vi "Defender_din_lorero.vi"(8 "IA State":T7={"our_robots"=[], "enemy_robots"=[], "balls"=[], "geometry"={"field_length"=0, "field_width"=0, "goal_width"=0, "goal_depth"=0, "center_circle_radius"=0, "defense_width"=0, "defense_depth"=0, "free_kick_from_defense_dist"=0, "penalty_spot_from_field_line_dist"=0, "penalty_line_from_spot_dist"=0, "half_moon_depth"=0, "half_moon_width"=0}, "IA Judge"={"stage"="", "command"="", "our_goalie_id"=0.0, "enemy_goalie_id"=0.0, "command enum"=enum."Halt", "Time"=enum."Azul"}, "Received Timestamp"=timestamp(0 s since 1904-01-01), "Events"={"Touch"=FALSE, "id touch"=0.0, "Ball out of \nVision"=FALSE, "Ball inside \nGoalie area"=FALSE, "Robot not responding"=FALSE, "Robots responding status"=[1.0, 1.0, 1.0, 1.0, 1.0, 1.0], "Enemy Ball \nPossession"=FALSE, "Id ini Possession"=0.0, "Ball Possesion"=FALSE, "Id Possesion"=0.0, "Ball at\nour goal side"=FALSE, "Ball at\ntouchline"=FALSE, "Ball at\nenemy goal side"=FALSE}}, 10 "balls":T6[](array[typedef]), 11 "Robot in":T1) -> (1 "Robot out":T1)   [LabVIEW 2018]
uses:
  Core/AI Robot.ctl
  Functions Enum.ctl
  AttackerStates.ctl
  Path Planning/RRT/PathDests.ctl
  Path Planning/RRT/PathDest.ctl
  Core/AI Input.ctl
  Core/AI Ball.ctl
  Core/Field Size.ctl
  Core/AI Judge.ctl
  Command Enum.ctl
  Util/Events/Events.ctl
  <vilib>/Analysis/_algsub.llb/Real Vector Norm.vi
  <vilib>/Analysis/NI_AALPro.lvlib
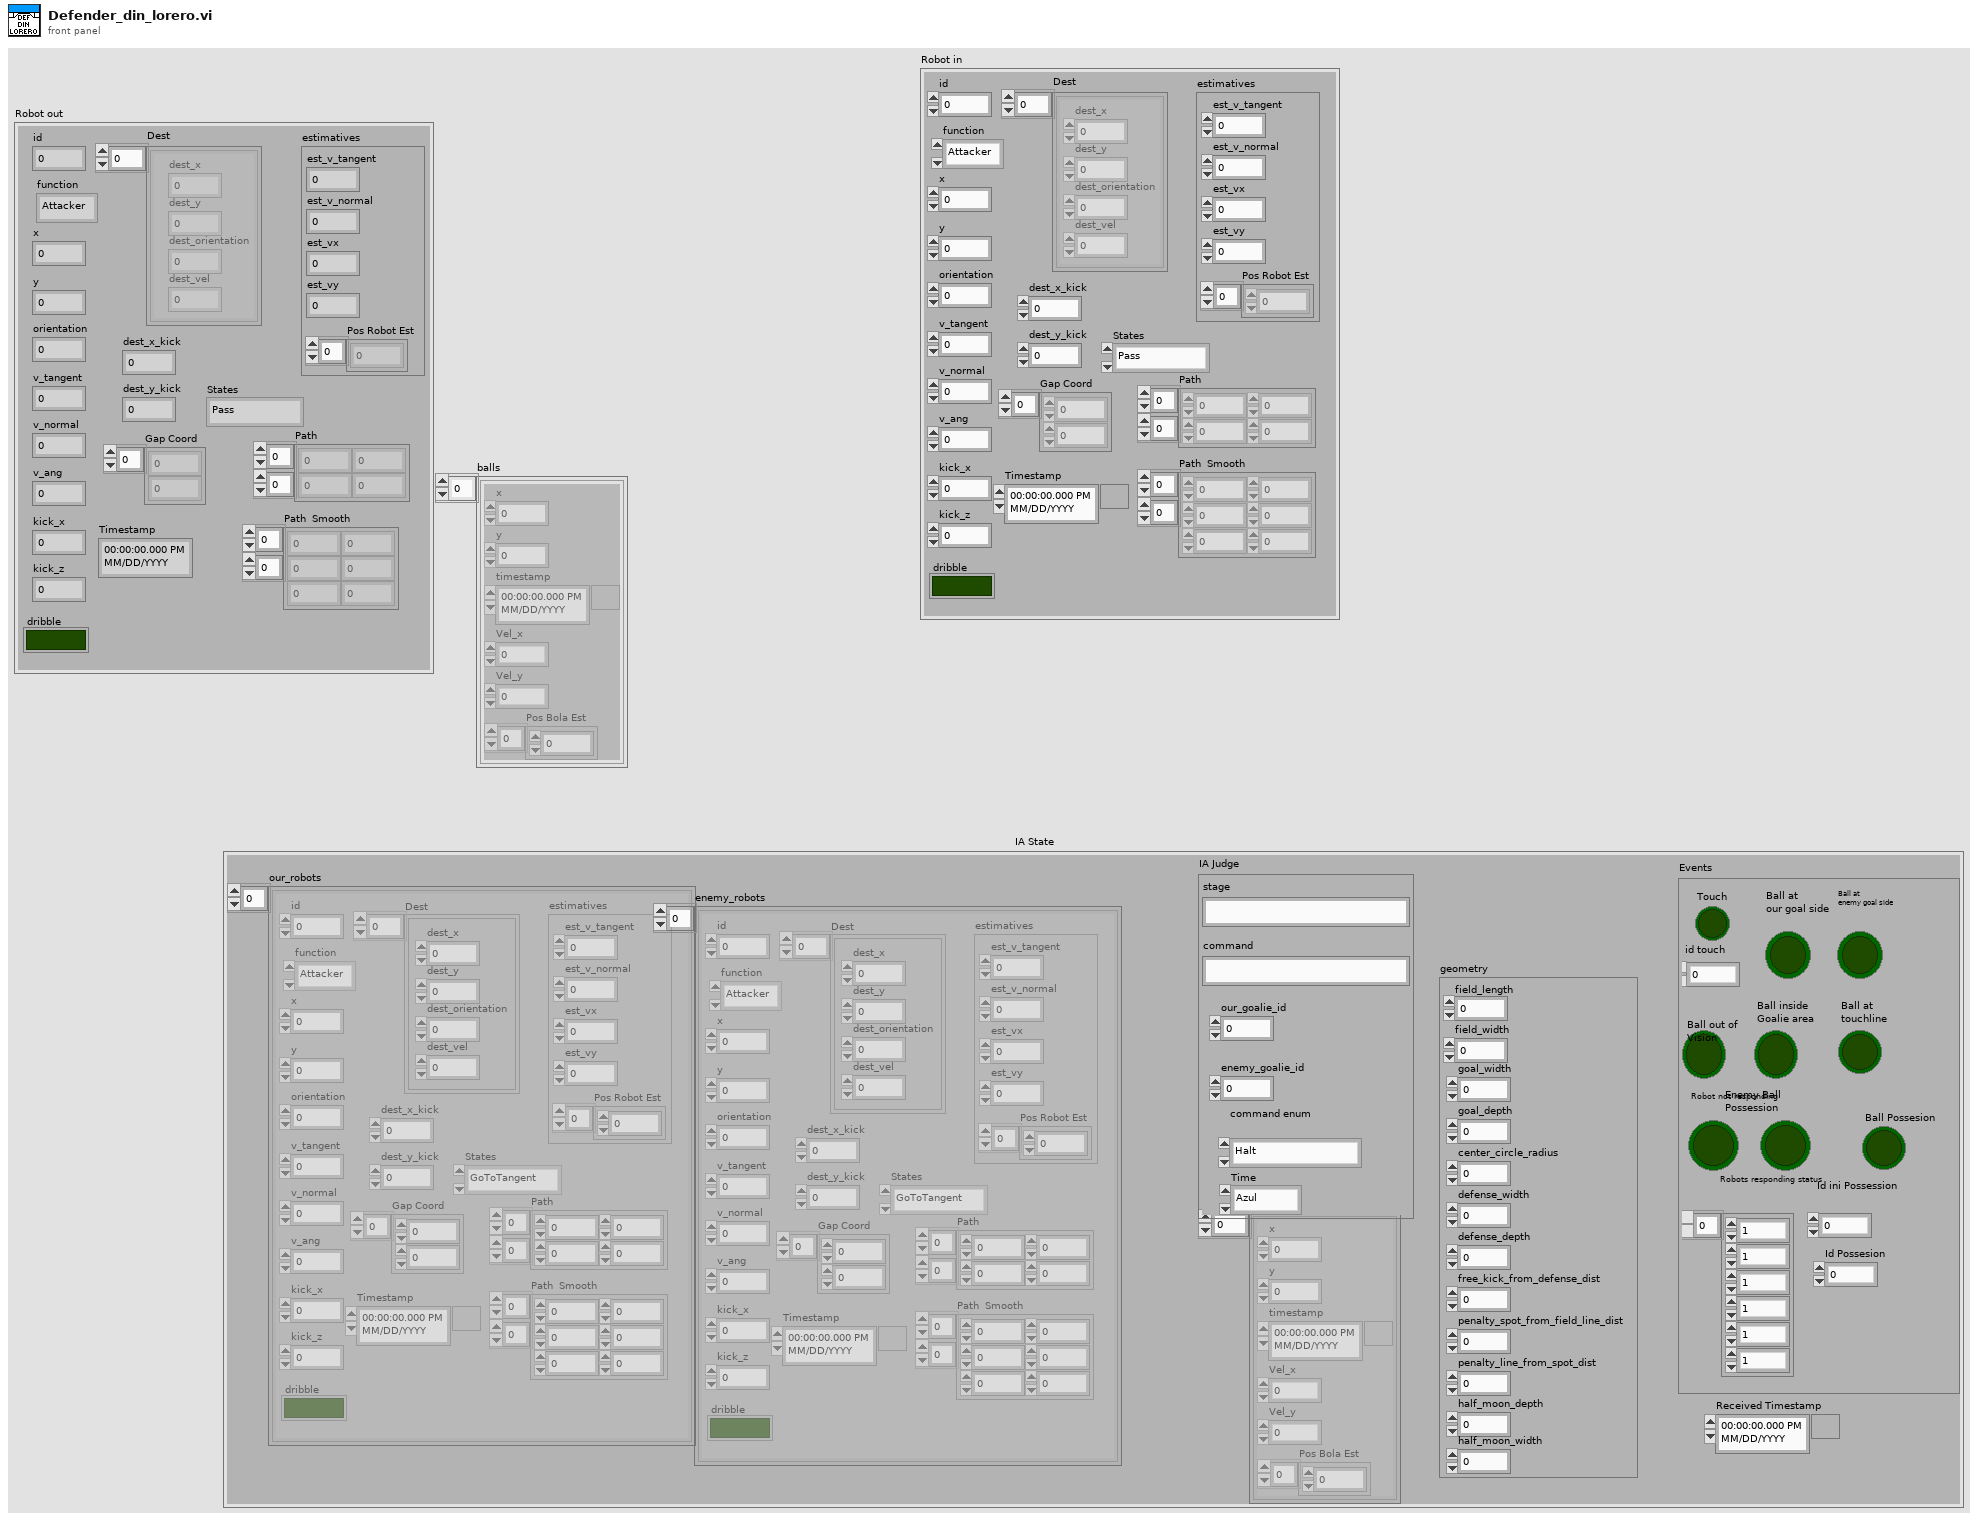
[diagram p1: front panel]
types:
  T1 = typedef "AI Robot.ctl" = cluster{"id":u32, "function":T2, "x":dbl, "y":dbl, "orientation":dbl, "v_tangent":dbl, "v_normal":dbl, "v_ang":dbl, "kick_x":dbl, "kick_z":dbl, "dribble":bool, "Timestamp":timestamp, "estimatives":cluster{"est_v_tangent":dbl, "est_v_normal":dbl, "est_vx":dbl, "est_vy":dbl, "Pos Robot Est":dbl[]}, "dest_x_kick":dbl, "dest_y_kick":dbl, "Gap Coord":dbl[], "States":T3, "Path ":dbl[][], "Path  Smooth":dbl[][], "Dest":T4}
  T2 = typedef "Functions Enum.ctl" = enum16{"Attacker", "Goalie", "Defender", "Striker", "Goto 0", "Dummy", "Kicker", "ZigZag"}
  T3 = typedef "AttackerStates.ctl" = enum16{"Pass", "GoToTangent", "BallGetting", "GoToKick", "Rotate anti-clockwise", "Rotate Clockwise", ""}
  T4 = typedef "PathDests.ctl" = T5[]
  T5 = typedef "PathDest.ctl" = cluster{"dest_x":dbl, "dest_y":dbl, "dest_orientation":dbl, "dest_vel":dbl}
  T6 = typedef "AI Ball.ctl" = cluster{"x":dbl, "y":dbl, "timestamp":timestamp, "Vel_x":dbl, "Vel_y":dbl, "Pos Bola Est":dbl[]}
  T7 = typedef "AI Input.ctl" = cluster{"our_robots":T1[], "enemy_robots":T1[], "balls":T6[], "geometry":T8, "IA Judge":T9, "Received Timestamp":timestamp, "Events":T11}
  T8 = typedef "Field Size.ctl" = cluster{"field_length":u32, "field_width":u32, "goal_width":u32, "goal_depth":u32, "center_circle_radius":u32, "defense_width":u32, "defense_depth":u32, "free_kick_from_defense_dist":u32, "penalty_spot_from_field_line_dist":u32, "penalty_line_from_spot_dist":u32, "half_moon_depth":u32, "half_moon_width":u32}
  T9 = typedef "AI Judge.ctl" = cluster{"stage":string, "command":string, "our_goalie_id":dbl, "enemy_goalie_id":dbl, "command enum":T10, "Time":enum16{"Azul", "Amarelo"}}
  T10 = typedef "Command Enum.ctl" = enum16{"Halt", "Stop", "Force Start", "PKA Normal Start", "Prepare Kickoff Ally", "PKE Normal Start", "Prepare Kickoff Enemy", "Prepare Penalty Ally", "PPA Normal Start", "Prepare Penalty Enemy", "PPE Normal Start", "Ball Placement Enemy Up", "Ball Placement Enemy Down", "Ball Placement Ally Up", "Ball Placement Ally Mid", "Ball Placement Ally Down", "Indirect Free Enemy", "Indirect Free Ally", "Timeout Enemy", "Timeout Ally", "Goal Enemy", "Goal Ally", "Normal Half Time", "Extra Time Break", "Extra Half Time", "None", "Post Game"}
  T11 = typedef "Events.ctl" = cluster{"Touch":bool, "id touch":dbl, "Ball out of \nVision":bool, "Ball inside \nGoalie area":bool, "Robot not responding":bool, "Robots responding status":dbl[], "Enemy Ball \nPossession":bool, "Id ini Possession":dbl, "Ball Possesion":bool, "Id Possesion":dbl, "Ball at\nour goal side":bool, "Ball at\ntouchline":bool, "Ball at\nenemy goal side":bool}
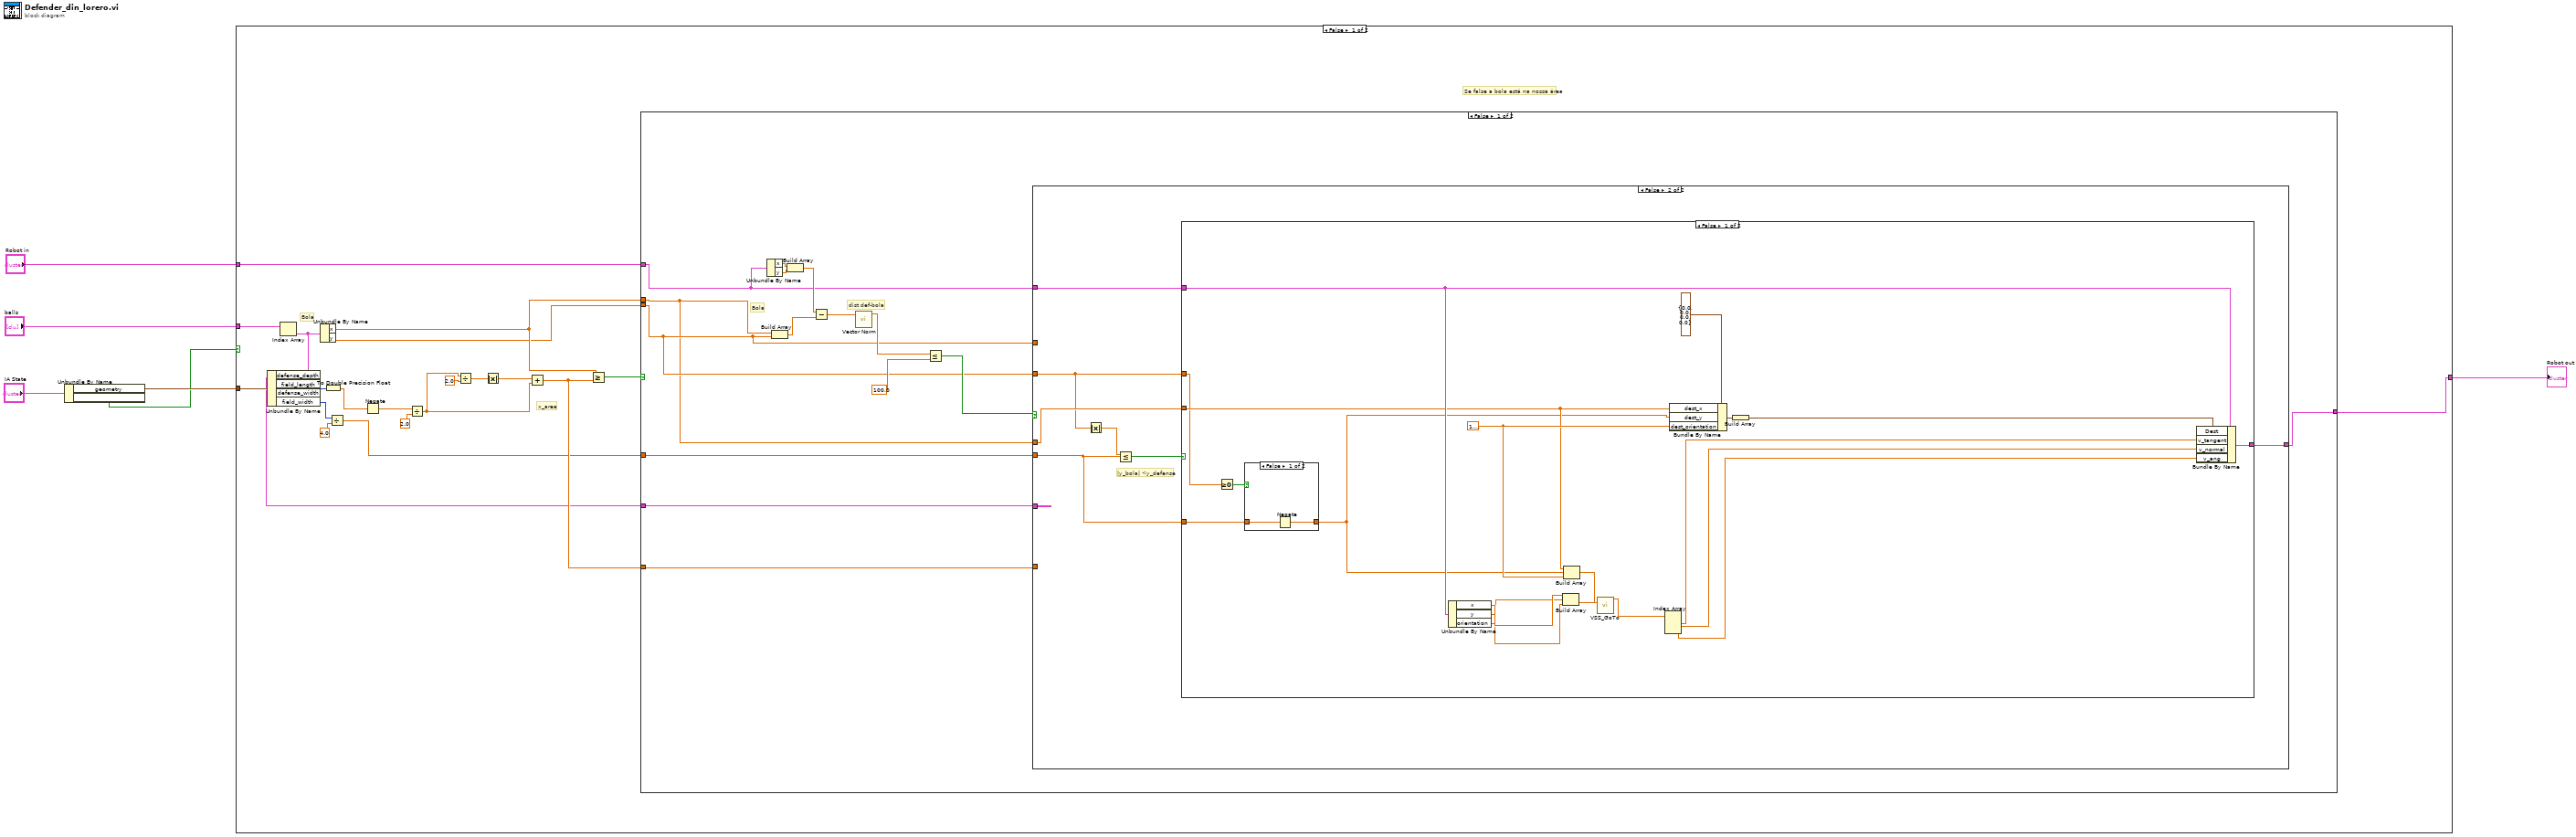
[diagram p0: block diagram]
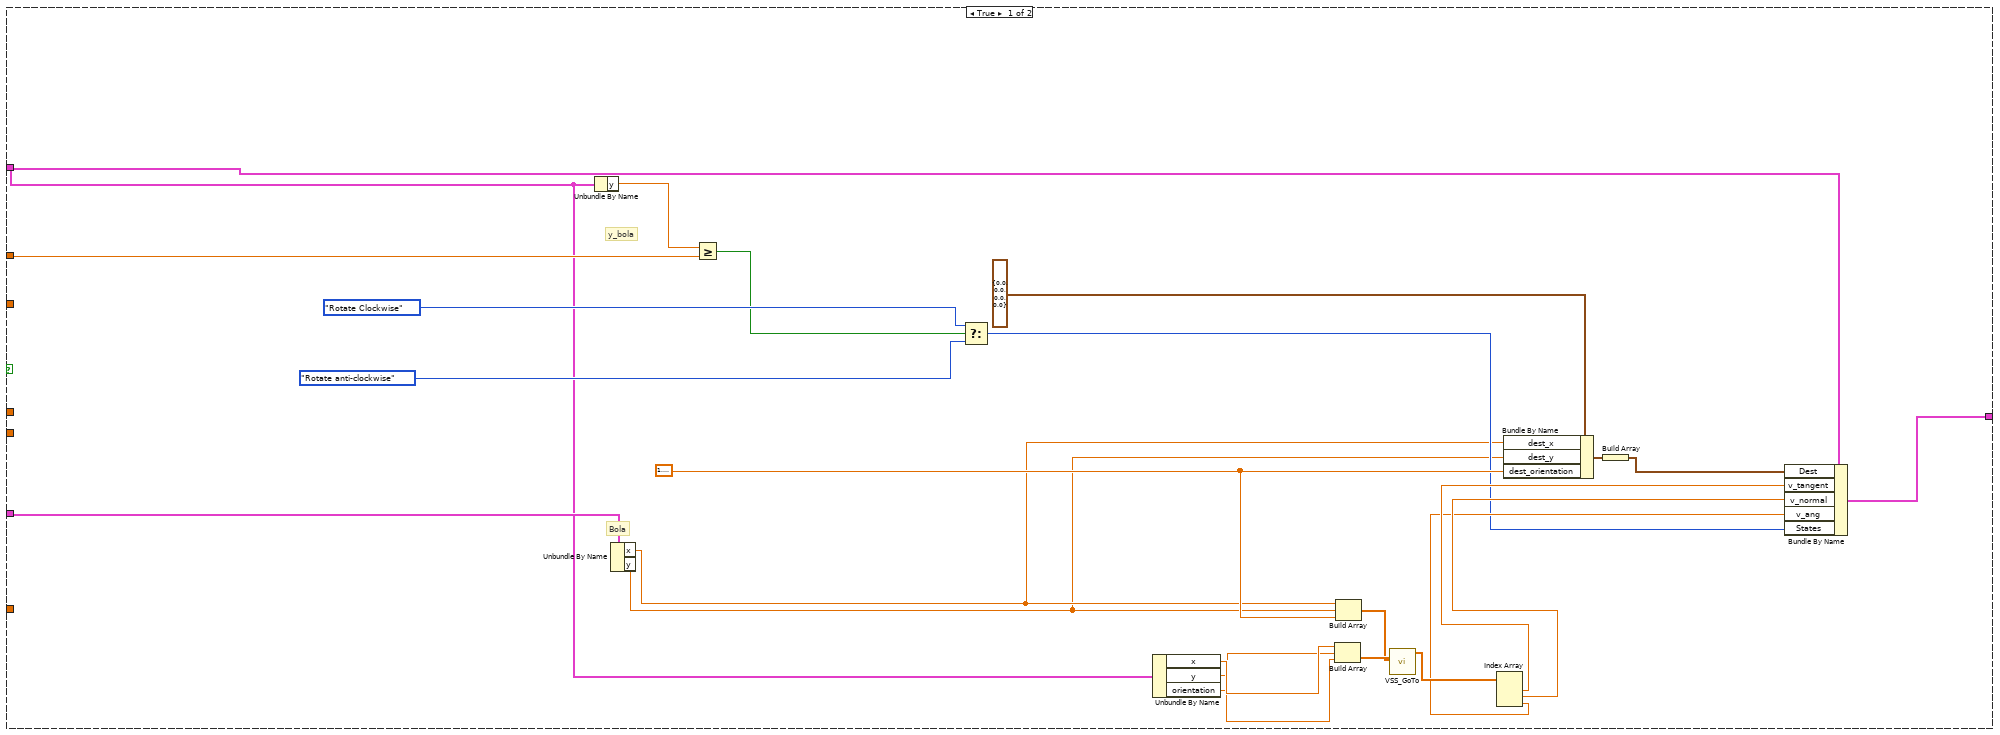
[diagram p2: hidden frame]
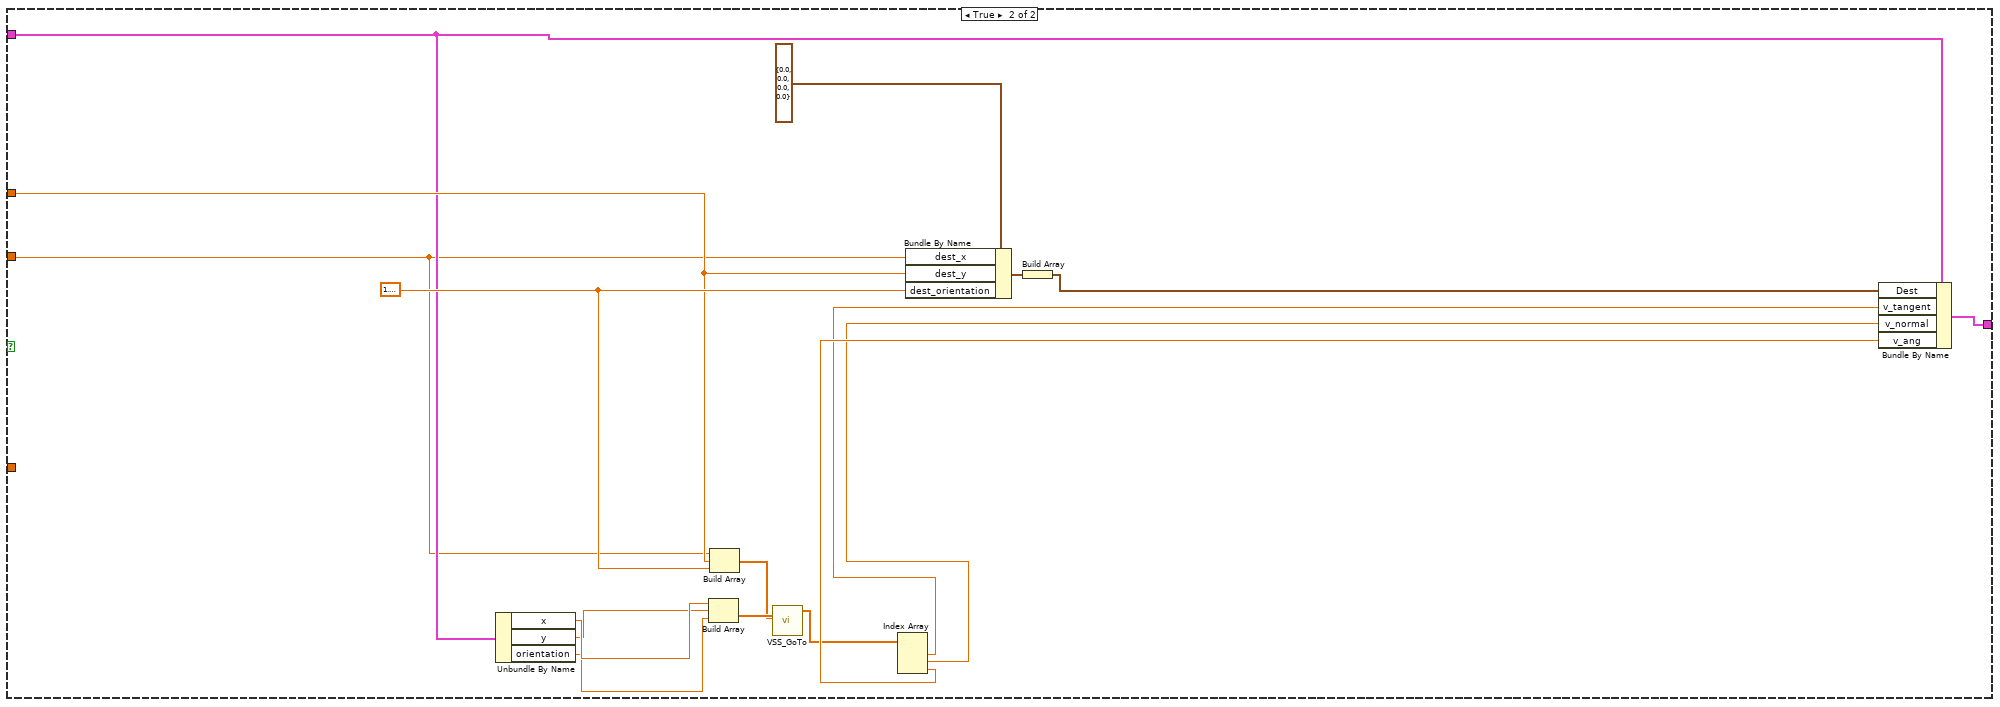
[diagram p4: hidden frame]
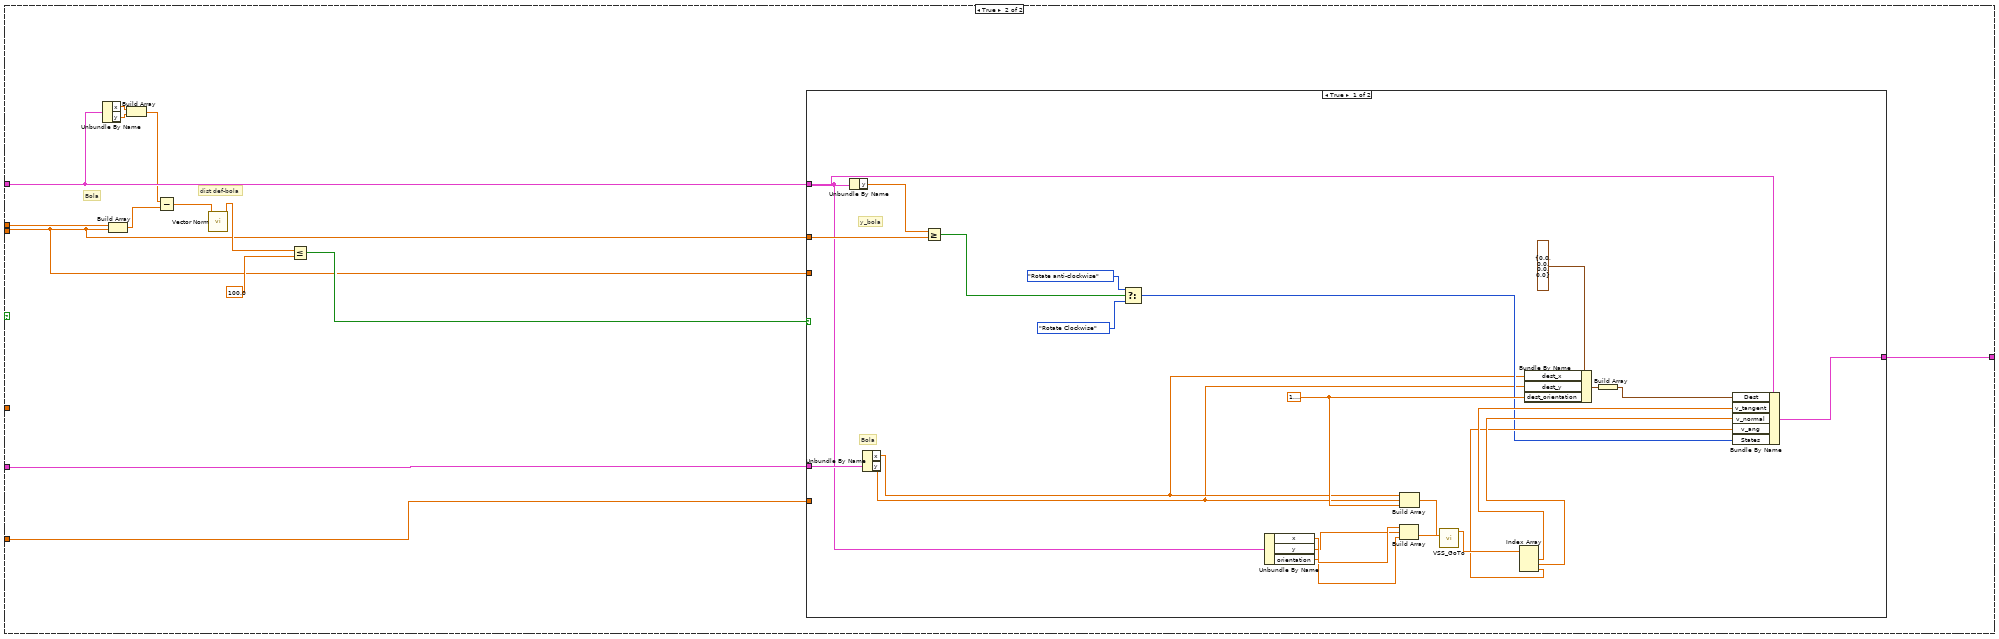
[diagram p5: hidden frame]
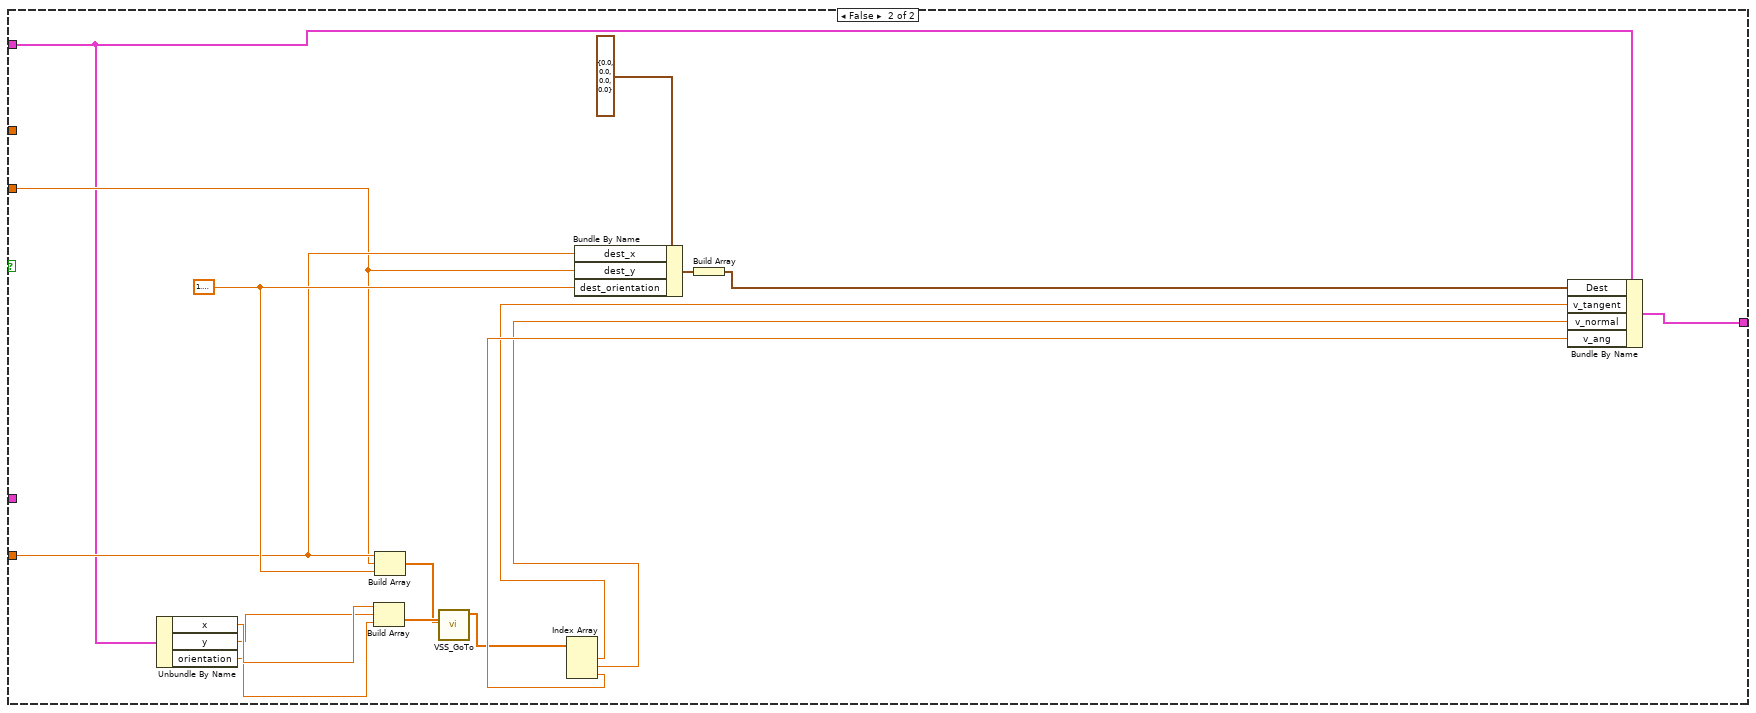
[diagram p6: hidden frame]
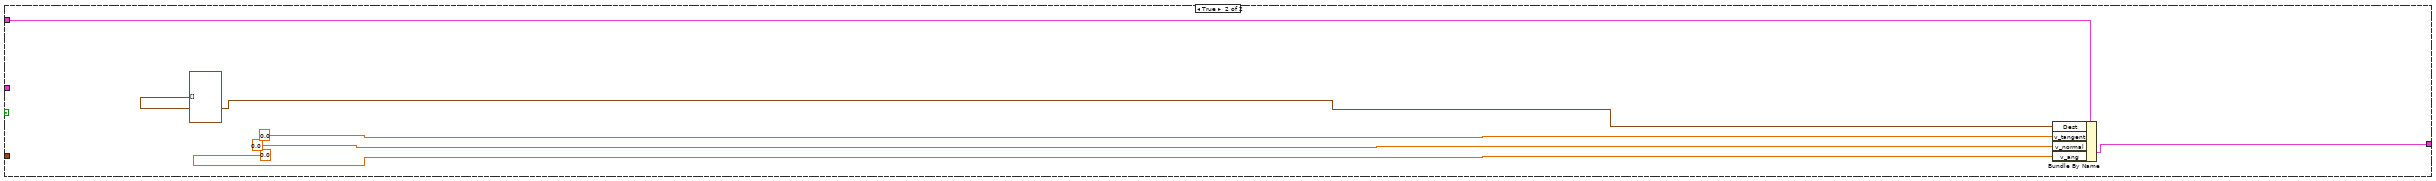
[diagram p7: hidden frame]
diagram:
  n1 = Unbundle By Name("IA State") -> ("geometry"=w3:T8, "Events.Ball out of \nVision"=w2:bool)
  n2 = case shown="False" w2 {
    tunnel: "Robot in" -> [w19 w169]
    tunnel: [w17 w168] -> w4
    tunnel: w3 -> [w25 _]
    tunnel: "balls" -> [w26 _]
    frame False {
      # "Se false a bola está na nossa área"
      # "x_area"
      # "Bola"
      n3 = Unbundle By Name(w25) -> ("field_length"=w23:u32, "field_width"=w10:u32)  [unwired: 2 out]
      n4 = Index Array(array=w26) -> (element=w14:T6)  [unwired: 1 in]
      n5 = Unbundle By Name(w14) -> ("x"=w16:dbl, "y"=w15:dbl)
      n6 = To Double Precision Float(number=w23) -> (double precision float=w22:dbl)
      n7 = Divide(x=w10, y=4.0) -> (x/y=w9:dbl)
      n8 = Negate(x=w22) -> (-x=w21:dbl)
      n9 = Divide(x=w21, y=2.0) -> (x/y=w12:dbl)
      n10 = Divide(x=w12, y=2.0) -> (x/y=w8:dbl)
      n11 = Absolute Value(x=w8) -> (abs(x)=w7:dbl)
      n12 = Add(x=w7, y=w12) -> (x+y=w18:dbl)
      n13 = Greater Or Equal?(x=w16, y=w18) -> (x >= y?=w20:bool)
      n14 = case shown="False" w20 {
        tunnel: w19 -> [w33 w123]
        tunnel: w18 -> [w31 w126]
        tunnel: [w28 w125] -> w17
        tunnel: w16 -> [w29 w124]
        tunnel: w15 -> [w30 w113]
        tunnel: w14 -> [w32 w114]
        tunnel: w9 -> [w27 _]
        frame False {
          # "dist def-bola"
          # "Bola"
          n15 = Unbundle By Name(w33) -> ("x"=w41:dbl, "y"=w40:dbl)
          n16 = Build Array(w29, w30) -> (w38:dbl[])
          n17 = Build Array(w41, w40) -> (w39:dbl[])
          n18 = Subtract(x=w39, y=w38) -> (x-y=w37:dbl[])
          n19 = call-poly <vilib>:"Vector Norm.vi"("Input Vector"=w37) -> ("norm"=w36:dbl)  [unwired: 9 in, 1 out]
          n20 = Less Or Equal?(x=w36, y=100.0) -> (x <= y?=w34:bool)
          n21 = case shown="False" w34 {
            tunnel: w31 -> [_ _]
            tunnel: w30 -> [_ w69]
            tunnel: w33 -> [w43 w72]
            tunnel: [w42 w71] -> w28
            tunnel: w30 -> [w64 _]
            tunnel: w32 -> [w46 _]
            tunnel: w29 -> [_ w70]
            tunnel: w27 -> [_ w66]
            frame True {
              w53 = 1.5707963267948966
              # "Bola"
              # "y_bola"
              n22 = Unbundle By Name(w43) -> ("y"=w65:dbl)
              n23 = Unbundle By Name(w46) -> ("x"=w45:dbl, "y"=w44:dbl)
              n24 = Greater Or Equal?(x=w65, y=w64) -> (x >= y?=w61:bool)
              n25 = Select(t=AttackerStates."Rotate Clockwise" ("States"), s=w61, f=AttackerStates."Rotate anti-clockwise" ("States")) -> (s? t:f=w47:T3)
              n26 = Unbundle By Name(w43) -> ("x"=w58:dbl, "y"=w56:dbl, "orientation"=w57:dbl)
              n27 = Build Array(w58, w56, w57) -> (w54:dbl[])
              n28 = Build Array(w45, w44, w53) -> (w52:dbl[])
              n29 = call "VSS_GoTo.vi"("SetPoint"=w52, "Position"=w54) -> ("Output Vel"=w55:dbl[])  [unwired: 9 in]
              n30 = Index Array(array=w55) -> (element #1=w50:dbl, element #2=w49:dbl, element #3=w48:dbl)  [unwired: 3 in]
              n31 = Bundle By Name(cluster=T5 {"dest_x"=0.0, "dest_y"=0.0, "dest_orientation"=0.0, "dest_vel"=0.0} ("element"), "dest_x"=w45, "dest_y"=w44, "dest_orientation"=w53) -> (w59:T5)
              n32 = Build Array(w59) -> (w51:T5[])
              n33 = Bundle By Name(cluster=w43, "Dest"=w51, "v_tangent"=w50, "v_normal"=w49, "v_ang"=w48, "States"=w47) -> (w42:T1)
            }
            frame False {
              # "|y_bola| <y_defense"
              n34 = Absolute Value(x=w69) -> (abs(x)=w68:dbl)
              n35 = Less Or Equal?(x=w68, y=w66) -> (x <= y?=w67:bool)
              n36 = case shown="False" w67 {
                tunnel: w69 -> [w76 w100]
                tunnel: w72 -> [w79 w98]
                tunnel: [w78 w97] -> w71
                tunnel: w70 -> [w77 w96]
                tunnel: w66 -> [w74 _]
                frame False {
                  w81 = 1.5707963267948966
                  n37 = Greater Or Equal To 0?(x=w76) -> (x >= 0?=w75:bool)
                  n38 = case shown="False" w75 {
                    tunnel: w74 -> [w94 w95]
                    tunnel: [w93 w95] -> w73
                    frame False {
                      n39 = Negate(x=w94) -> (-x=w93:dbl)
                    }
                    frame True {
                    }
                  }
                  n40 = Unbundle By Name(w79) -> ("x"=w87:dbl, "y"=w85:dbl, "orientation"=w86:dbl)
                  n41 = Build Array(w87, w85, w86) -> (w82:dbl[])
                  n42 = Build Array(w77, w73, w81) -> (w80:dbl[])
                  n43 = call "VSS_GoTo.vi"("SetPoint"=w80, "Position"=w82) -> ("Output Vel"=w83:dbl[])  [unwired: 9 in]
                  n44 = Index Array(array=w83) -> (element #1=w91:dbl, element #2=w84:dbl, element #3=w92:dbl)  [unwired: 3 in]
                  n45 = Bundle By Name(cluster=T5 {"dest_x"=0.0, "dest_y"=0.0, "dest_orientation"=0.0, "dest_vel"=0.0} ("element"), "dest_x"=w77, "dest_y"=w73, "dest_orientation"=w81) -> (w88:T5)
                  n46 = Build Array(w88) -> (w90:T5[])
                  n47 = Bundle By Name(cluster=w79, "Dest"=w90, "v_tangent"=w91, "v_normal"=w84, "v_ang"=w92) -> (w78:T1)
                }
                frame True {
                  w101 = 1.5707963267948966
                  n48 = Unbundle By Name(w98) -> ("x"=w107:dbl, "y"=w105:dbl, "orientation"=w106:dbl)
                  n49 = Build Array(w107, w105, w106) -> (w102:dbl[])
                  n50 = Build Array(w96, w100, w101) -> (w99:dbl[])
                  n51 = call "VSS_GoTo.vi"("SetPoint"=w99, "Position"=w102) -> ("Output Vel"=w103:dbl[])  [unwired: 9 in]
                  n52 = Index Array(array=w103) -> (element #1=w111:dbl, element #2=w104:dbl, element #3=w112:dbl)  [unwired: 3 in]
                  n53 = Bundle By Name(cluster=T5 {"dest_x"=0.0, "dest_y"=0.0, "dest_orientation"=0.0, "dest_vel"=0.0} ("element"), "dest_x"=w96, "dest_y"=w100, "dest_orientation"=w101) -> (w108:T5)
                  n54 = Build Array(w108) -> (w110:T5[])
                  n55 = Bundle By Name(cluster=w98, "Dest"=w110, "v_tangent"=w111, "v_normal"=w104, "v_ang"=w112) -> (w97:T1)
                }
              }
            }
          }
        }
        frame True {
          # "dist def-bola"
          # "Bola"
          n56 = Unbundle By Name(w123) -> ("x"=w122:dbl, "y"=w121:dbl)
          n57 = Build Array(w124, w113) -> (w119:dbl[])
          n58 = Build Array(w122, w121) -> (w120:dbl[])
          n59 = Subtract(x=w120, y=w119) -> (x-y=w118:dbl[])
          n60 = call-poly <vilib>:"Vector Norm.vi"("Input Vector"=w118) -> ("norm"=w117:dbl)  [unwired: 9 in, 1 out]
          n61 = Less Or Equal?(x=w117, y=100.0) -> (x <= y?=w115:bool)
          n62 = case shown="True" w115 {
            tunnel: w126 -> [_ w155]
            tunnel: w113 -> [_ w154]
            tunnel: w123 -> [w128 w152]
            tunnel: [w127 w151] -> w125
            tunnel: w113 -> [w149 _]
            tunnel: w114 -> [w131 _]
            frame True {
              w138 = 1.5707963267948966
              # "Bola"
              # "y_bola"
              n63 = Unbundle By Name(w128) -> ("y"=w150:dbl)
              n64 = Unbundle By Name(w131) -> ("x"=w130:dbl, "y"=w129:dbl)
              n65 = Greater Or Equal?(x=w150, y=w149) -> (x >= y?=w146:bool)
              n66 = Select(t=AttackerStates."Rotate anti-clockwise" ("States"), s=w146, f=AttackerStates."Rotate Clockwise" ("States")) -> (s? t:f=w132:T3)
              n67 = Unbundle By Name(w128) -> ("x"=w143:dbl, "y"=w141:dbl, "orientation"=w142:dbl)
              n68 = Build Array(w143, w141, w142) -> (w139:dbl[])
              n69 = Build Array(w130, w129, w138) -> (w137:dbl[])
              n70 = call "VSS_GoTo.vi"("SetPoint"=w137, "Position"=w139) -> ("Output Vel"=w140:dbl[])  [unwired: 9 in]
              n71 = Index Array(array=w140) -> (element #1=w135:dbl, element #2=w134:dbl, element #3=w133:dbl)  [unwired: 3 in]
              n72 = Bundle By Name(cluster=T5 {"dest_x"=0.0, "dest_y"=0.0, "dest_orientation"=0.0, "dest_vel"=0.0} ("element"), "dest_x"=w130, "dest_y"=w129, "dest_orientation"=w138) -> (w144:T5)
              n73 = Build Array(w144) -> (w136:T5[])
              n74 = Bundle By Name(cluster=w128, "Dest"=w136, "v_tangent"=w135, "v_normal"=w134, "v_ang"=w133, "States"=w132) -> (w127:T1)
            }
            frame False {
              w156 = 1.5707963267948966
              n75 = Unbundle By Name(w152) -> ("x"=w162:dbl, "y"=w160:dbl, "orientation"=w161:dbl)
              n76 = Build Array(w162, w160, w161) -> (w157:dbl[])
              n77 = Build Array(w155, w154, w156) -> (w153:dbl[])
              n78 = call "VSS_GoTo.vi"("SetPoint"=w153, "Position"=w157) -> ("Output Vel"=w158:dbl[])  [unwired: 9 in]
              n79 = Index Array(array=w158) -> (element #1=w166:dbl, element #2=w159:dbl, element #3=w167:dbl)  [unwired: 3 in]
              n80 = Bundle By Name(cluster=T5 {"dest_x"=0.0, "dest_y"=0.0, "dest_orientation"=0.0, "dest_vel"=0.0} ("element"), "dest_x"=w155, "dest_y"=w154, "dest_orientation"=w156) -> (w163:T5)
              n81 = Build Array(w163) -> (w165:T5[])
              n82 = Bundle By Name(cluster=w152, "Dest"=w165, "v_tangent"=w166, "v_normal"=w159, "v_ang"=w167) -> (w151:T1)
            }
          }
        }
      }
    }
    frame True {
      n83 = Bundle By Name(cluster=w169, "Dest"=T5[] [], "v_tangent"=0.0, "v_normal"=0.0, "v_ang"=0.0) -> (w168:T1)
    }
  }
  "Robot out" <- w4
